vi "GetGrowInfo.vi"(0 "XRef":T7, 1 "State In":T6) -> (14 "Grow Info":T2, 15 "Fatal Error Out":T1)   [LabVIEW 2021, in "FirstXNode .xnode"]
uses:
  FirstXNode .xnode
  <vilib>/XNodeSupport/XNodeXNodeRef.ctl
  State.ctl
  <vilib>/XNodeSupport/XNodeBounds.ctl
  <vilib>/XNodeSupport/XNodeInt.ctl
  <vilib>/XNodeSupport/XNodeGrowInfo.ctl
  <vilib>/XNodeSupport/XNodeBool.ctl
  <vilib>/XNodeSupport/XNodeErrorCluster.ctl
  <vilib>/XNodeSupport/NI_XNodeSupport.lvlib
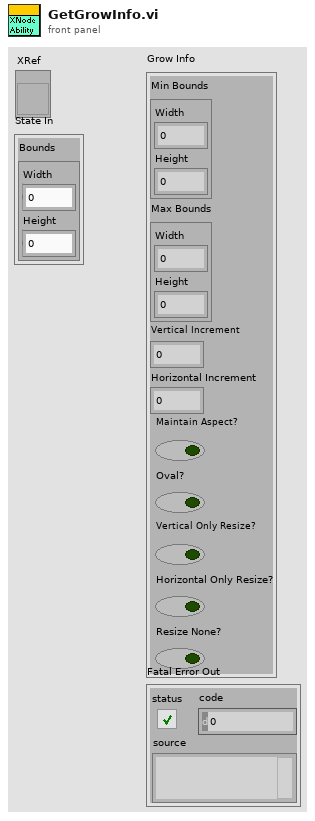
[diagram p1: front panel]
types:
  T1 = typedef "NI_XNodeSupport.lvlib/XNodeErrorCluster.ctl" = errorcluster
  T2 = typedef "NI_XNodeSupport.lvlib/XNodeGrowInfo.ctl" = cluster{"Min Bounds":T3, "Max Bounds":T3, "Vertical Increment":T4, "Horizontal Increment":T4, "Maintain Aspect?":T5, "Oval?":T5, "Vertical Only Resize?":T5, "Horizontal Only Resize?":T5, "Resize None?":T5}
  T3 = typedef "NI_XNodeSupport.lvlib/XNodeBounds.ctl" = cluster{"Width":T4, "Height":T4}
  T4 = typedef "NI_XNodeSupport.lvlib/XNodeInt.ctl" = i32
  T5 = typedef "NI_XNodeSupport.lvlib/XNodeBool.ctl" = bool
  T6 = typedef "FirstXNode .xnode/State.ctl" = cluster{"Bounds":T3}
  T7 = typedef "NI_XNodeSupport.lvlib/XNodeXNodeRef.ctl" = refnum<vi>
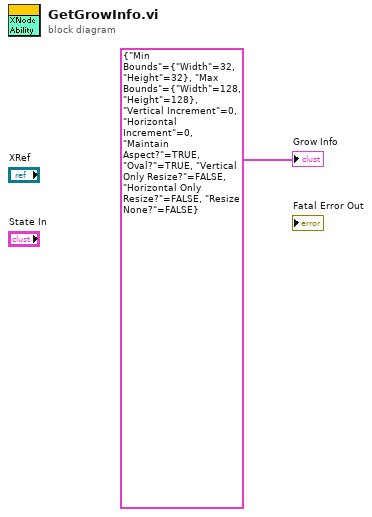
[diagram p0: block diagram]
diagram:
  "Grow Info" <- T2 {"Min Bounds"={"Width"=32, "Height"=32}, "Max Bounds"={"Width"=128, "Height"=128}, "Vertical Increment"=0, "Horizontal Increment"=0, "Maintain Aspect?"=TRUE, "Oval?"=TRUE, "Vertical Only Resize?"=FALSE, "Horizontal Only Resize?"=FALSE, "Resize None?"=FALSE} ("Grow Info")
